vi "Edge Detect.vi"(9 "edge (rising)":enum16{"rising", "falling"}(ring), 11 "signal in":bool) -> (3 "edge detected?":bool)   [LabVIEW 2013, in "I2S-TDM.lvlib"]
uses:
  I2S-TDM.lvlib
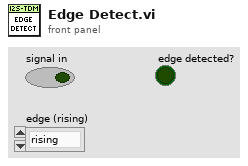
[diagram p1: front panel]
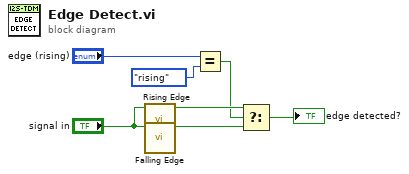
[diagram p0: block diagram]
diagram:
  n1 = call "Rising Edge.vi"("signal in"="signal in") -> ("rising edge?"=w3:bool)  [unwired: 10 in]
  n2 = call "Falling Edge.vi"("signal in"="signal in") -> ("falling edge?"=w4:bool)  [unwired: 10 in]
  n3 = Equal?(x="edge (rising)", y=enum16{"rising", "falling"}."rising" ("sync edge trigger")) -> (x = y?=w2:bool)
  n4 = Select(t=w3, s=w2, f=w4) -> (s? t:f=→"edge detected?":bool)
